vi "Limelight HatchPanel.vi"() -> ()   [LabVIEW 2018]
uses:
  <vilib>/Rock Robotics/Network Tables/NT Read Number.vi
panel:
  in  "allowed error":dbl=0.8
  in  "kpDist":dbl=0.2
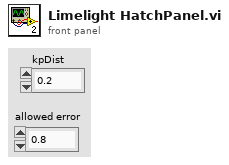
[diagram p1: front panel]
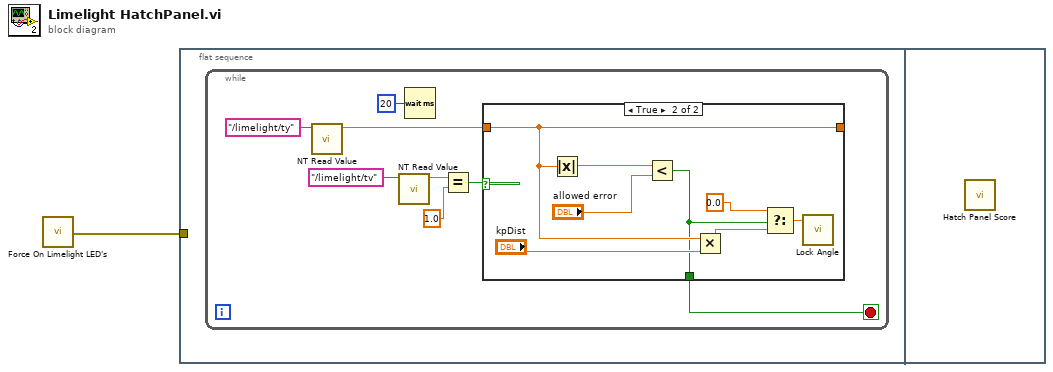
[diagram p0: block diagram]
diagram:
  n1 = call "Force On Limelight LED's.vi"() -> ("error out"=w1:errorcluster)  [unwired: 10 in]
  n2 = flat-sequence {
    tunnel: w1 -> [_]
    frame #0 {
      n3 = while {
        stop <- w2 stop-if-true
        n4 = call-poly <vilib>:"NT Read Value.vi"("Name"="/limelight/ty") -> ("Numeric"=w4:dbl)  [unwired: 9 in, 1 out]
        n5 = call-poly <vilib>:"NT Read Value.vi"("Name"="/limelight/tv") -> ("Numeric"=w8:dbl)  [unwired: 9 in, 1 out]
        n6 = Wait (ms)(milliseconds to wait=u32 20) -> ()  [unwired: 1 out]
        n7 = Equal?(x=w8, y=1.0) -> (x = y?=w6:bool)
        n8 = case shown="True" w6 {
          tunnel: [w10 w17] -> _
          tunnel: w4 -> [w10 w17]
          tunnel: [_ w11] -> w2
          frame False {
          }
          frame True {
            n9 = Absolute Value(x=w17) -> (abs(x)=w16:dbl)
            n10 = Less?(x=w16, y="allowed error") -> (x < y?=w11:bool)
            n11 = Multiply(x=w17, y="kpDist") -> (x*y=w14:dbl)
            n12 = Select(t=0.0, s=w11, f=w14) -> (s? t:f=w13:dbl)
            n13 = call "Lock Angle.vi"("Setpoint"=w13) -> ()  [unwired: 11 in]
          }
        }
      }
    }
    frame #1 {
      n14 = call "Hatch Panel Score.vi"() -> ()  [unwired: 11 in, 1 out]
    }
  }
